vi "I have broken VIs.vi"   [LabVIEW 2025, in "Queue Driver.lvlib"]
uses:
  Queue Driver.lvlib
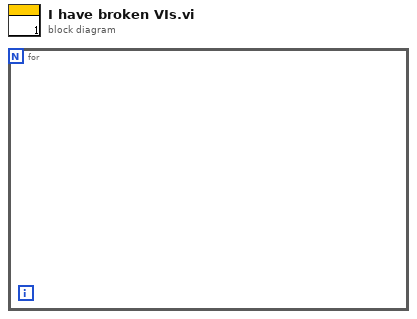
[diagram p0: block diagram]
diagram:
  n1 = for {
  }
